vi "Process_Traces.vi"(8 "Process data parameters in":T1={"Stop loop"={"Settings changed?"=FALSE, "Stop?"=refnum}, "Button refs"={"Stop program"=refnum, "Save settings"=refnum, "DAQ mode"=refnum, "Reset settings"=refnum, "Apply settings"=refnum, "Reset MAS"=refnum, "Reset SLV"=refnum, "Local DBase?"=refnum, "Last value DBase"=FALSE, "Database"=refnum, "Calibration"=refnum, "Save settings 2"=refnum}, "Process messages"={"Process message mode"=enum."Error", "Slave data?"=FALSE, "Length get settings message"=0, "Delta time"=0.0, "Data_Filter"={"Filter_Data"=FALSE, "Use_Thresh"=FALSE, "Reduce data?"=FALSE}, "Time_difference_stack"=[], "Starting sec"=0, "Ending sec"=0, "Ending sec 2"=0, "MAS_Page_Thresh"=refnum, "SLV_Page_Thresh"=refnum, "Database"=refnum}, "Settings state"={"MAS locked?"=refnum, "SLV locked?"=refnum}, "Mode"={"Mode"=enum."Dialog", "Expert?"=FALSE, "Dialog?"=FALSE}, "Alignment parameters"=refnum, "Timer parameters"=refnum, "Files"={"Path config file"=path "", "Path def. ini file"=path "", "Path ini file 1"=path "", "Path ini file 2"=path "", "Path RBF file"=path ""}, "Time difference"=refnum, "Alignment"={"GEN_Page_Calibrate"=refnum, "MAS_Page_Gain"=refnum, "MAS_Page_Offset"=refnum, "SLV_Page_Gain"=refnum, "SLV_Page_Offset"=refnum, "MAS_Page_Common"=refnum, "SLV_Page_Common"=refnum}, "Page Statistics"=refnum}, 9 "Length":i32, 10 "Data in":u8[](array[numeric]), 11 "Master?":bool=TRUE) -> (1 "Cut off":i16[](array[numeric]), 2 "Data out":u8[](array[numeric]), 3 "Offset":i16[](array[numeric]))   [LabVIEW 2013]
uses:
  Controls/Stop_Loop.ctl
  Controls/Button_Refs.ctl
  Controls/Process_Message_Mode.ctl
  Controls/Process_Messages.ctl
  Controls/Settings_State.ctl
  Controls/Mode.ctl
  Controls/Files.ctl
  Controls/Process_Data_Parameters.ctl
  Controls/Page_Calibration.ctl
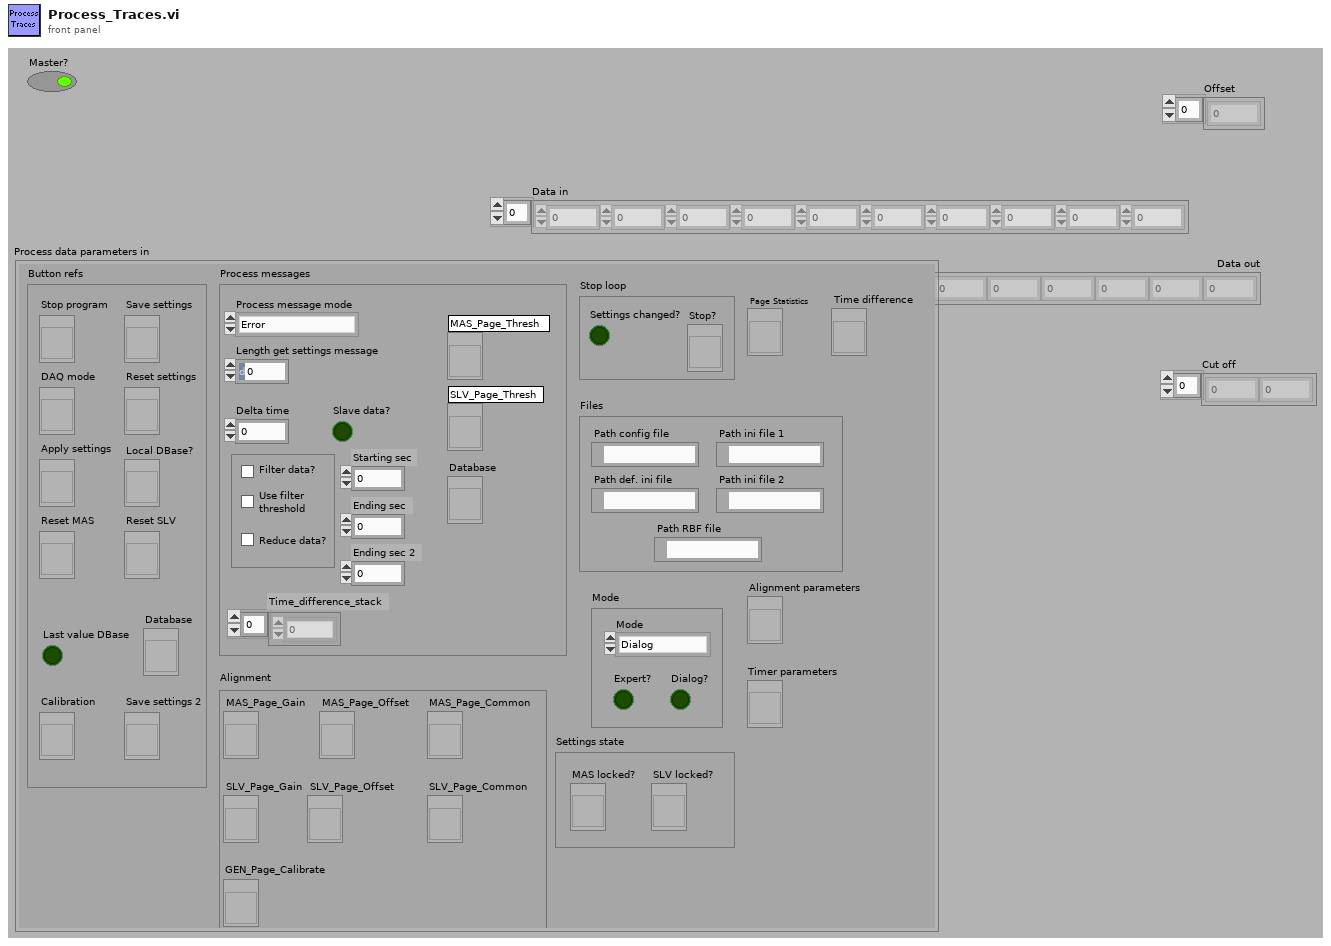
[diagram p1: front panel]
types:
  T1 = typedef "Process_Data_Parameters.ctl" = cluster{"Stop loop":T2, "Button refs":T3, "Process messages":T4, "Settings state":T6, "Mode":T7, "Alignment parameters":refnum<vi>, "Timer parameters":refnum<vi>, "Files":T8, "Time difference":refnum<vi>, "Alignment":T9, "Page Statistics":refnum<vi>}
  T2 = typedef "Stop_Loop.ctl" = cluster{"Settings changed?":bool, "Stop?":refnum<vi>}
  T3 = typedef "Button_Refs.ctl" = cluster{"Stop program":refnum<vi>, "Save settings":refnum<vi>, "DAQ mode":refnum<vi>, "Reset settings":refnum<vi>, "Apply settings":refnum<vi>, "Reset MAS":refnum<vi>, "Reset SLV":refnum<vi>, "Local DBase?":refnum<vi>, "Last value DBase":bool, "Database":refnum<vi>, "Calibration":refnum<vi>, "Save settings 2":refnum<vi>}
  T4 = typedef "Process_Messages.ctl" = cluster{"Process message mode":T5, "Slave data?":bool, "Length get settings message":i32, "Delta time":dbl, "Data_Filter":cluster{"Filter_Data":bool, "Use_Thresh":bool, "Reduce data?":bool}, "Time_difference_stack":u64[], "Starting sec":u64, "Ending sec":u64, "Ending sec 2":u64, "MAS_Page_Thresh":refnum<vi>, "SLV_Page_Thresh":refnum<vi>, "Database":refnum<vi>}
  T5 = typedef "Process_Message_Mode.ctl" = enum16{"Error", "Measurement data", "Comparator data", "One Second"}
  T6 = typedef "Settings_State.ctl" = cluster{"MAS locked?":refnum<vi>, "SLV locked?":refnum<vi>}
  T7 = typedef "Mode.ctl" = cluster{"Mode":enum8{"Stop", "Dialog", "Hisparc II", "Hisparc II DAQ", "Alignment"}, "Expert?":bool, "Dialog?":bool}
  T8 = typedef "Files.ctl" = cluster{"Path config file":path, "Path def. ini file":path, "Path ini file 1":path, "Path ini file 2":path, "Path RBF file":path}
  T9 = typedef "Page_Calibration.ctl" = cluster{"GEN_Page_Calibrate":refnum<vi>, "MAS_Page_Gain":refnum<vi>, "MAS_Page_Offset":refnum<vi>, "SLV_Page_Gain":refnum<vi>, "SLV_Page_Offset":refnum<vi>, "MAS_Page_Common":refnum<vi>, "SLV_Page_Common":refnum<vi>}
  T10 = cluster{"Filter_Data":bool, "Use_Thresh":bool, "Reduce data?":bool}
  T11 = cluster{"Ch1_Thres_Low":dbl, "Ch1_Thres_High":dbl, "Ch2_Thres_Low":dbl, "Ch2_Thres_High":dbl}
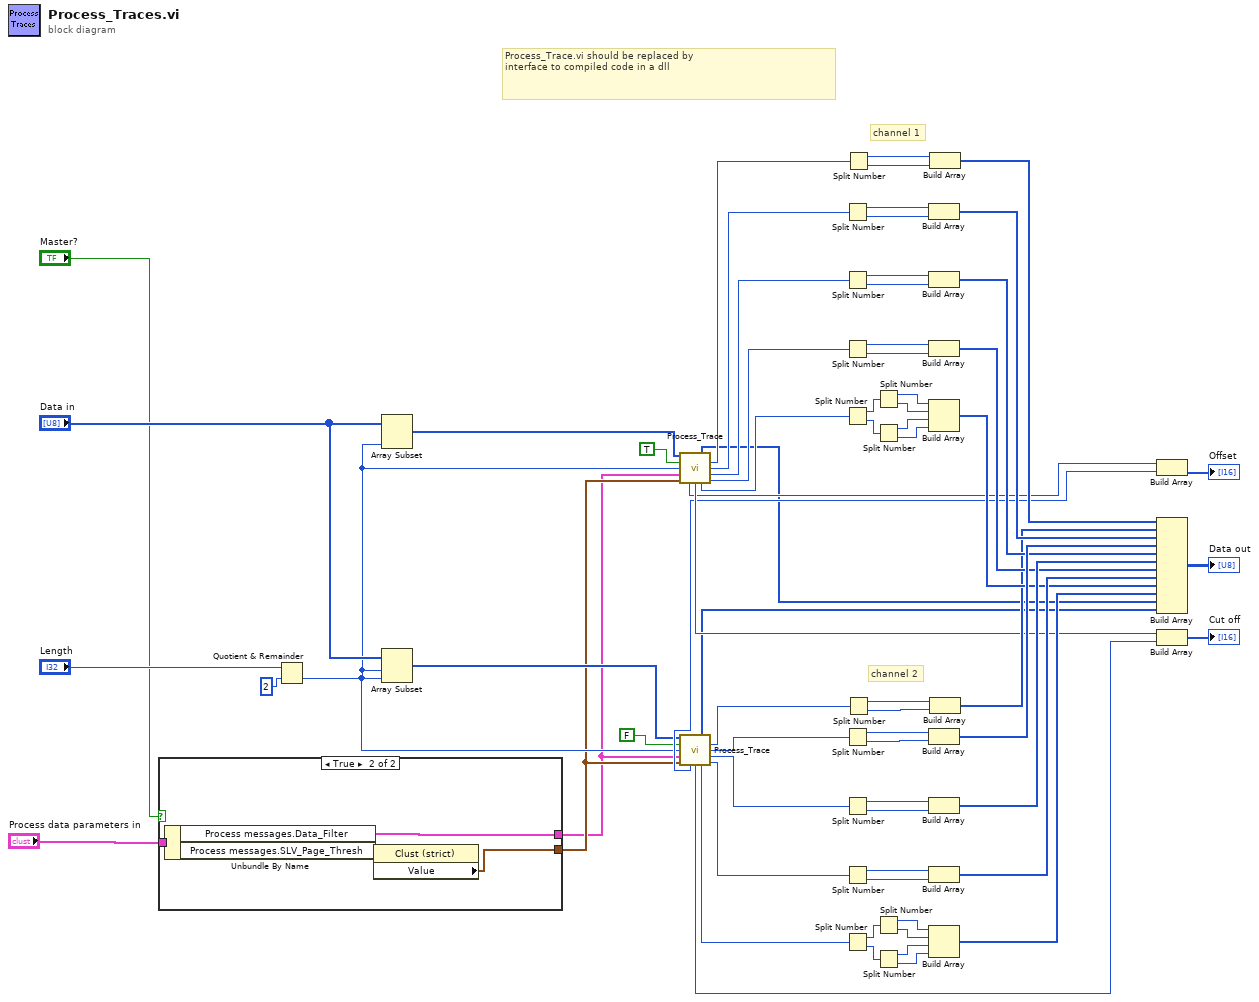
[diagram p0: block diagram]
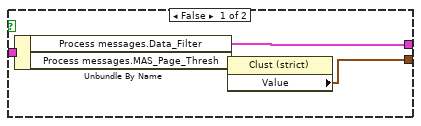
[diagram p2: hidden frame]
diagram:
  # "channel 1"
  # "channel 2"
  # "Process_Trace.vi should be replaced by\ninterface to compiled code in a dll"
  n1 = case shown="True" "Master?" {
    tunnel: "Process data parameters in" -> [w73 w77]
    tunnel: [w70 w74] -> w5
    tunnel: [w72 w76] -> w4
    frame False {
      n2 = Unbundle By Name(w73) -> ("Process messages.Data_Filter"=w72:T10, "Process messages.MAS_Page_Thresh"=w71:refnum<vi>)
      n3 = property class="Clust (strict)"(reference=w71) -> ("Value"=w70:T11)  [unwired: 1 in, 2 out]
    }
    frame True {
      n4 = Unbundle By Name(w77) -> ("Process messages.Data_Filter"=w76:T10, "Process messages.SLV_Page_Thresh"=w75:refnum<vi>)
      n5 = property class="Clust (strict)"(reference=w75) -> ("Value"=w74:T11)  [unwired: 1 in, 2 out]
    }
  }
  n6 = Quotient & Remainder(x="Length", y=2) -> (floor(x/y)=w8:i32)  [unwired: 1 out]
  n7 = Array Subset(array="Data in", length=w8) -> (w10:u8[])  [unwired: 1 in]
  n8 = Array Subset(array="Data in", index=w8, length=w8) -> (w9:u8[])
  n9 = call "Process_Trace.vi"("Data in"=w10, "Channel 1?"=TRUE, "Length"=w8, "Data_Filter"=w4, "M-Thresholds"=w5) -> ("Data out (8 bits)"=w1:u8[], "Standard deviation"=w24:i16, "Baseline"=w22:i16, "Number of peaks"=w20:i16, "Offset"=w12:i16, "Cut off"=w14:i16, "Integral"=w16:i32, "Pulse height"=w18:i16)  [unwired: 1 in, 2 out]
  n10 = call "Process_Trace.vi"("Data in"=w9, "Channel 1?"=FALSE, "Length"=w8, "Data_Filter"=w4, "M-Thresholds"=w5) -> ("Data out (8 bits)"=w2:u8[], "Standard deviation"=w23:i16, "Baseline"=w21:i16, "Number of peaks"=w19:i16, "Offset"=w11:i16, "Cut off"=w13:i16, "Integral"=w15:i32, "Pulse height"=w17:i16)  [unwired: 1 in, 2 out]
  n11 = Split Number(x=w22) -> (hi(x)=w40:u8, lo(x)=w39:u8)
  n12 = Split Number(x=w20) -> (hi(x)=w38:u8, lo(x)=w37:u8)
  n13 = Split Number(x=w18) -> (hi(x)=w36:u8, lo(x)=w35:u8)
  n14 = Split Number(x=w16) -> (hi(x)=w60:u16, lo(x)=w59:u16)
  n15 = Split Number(x=w21) -> (hi(x)=w46:u8, lo(x)=w45:u8)
  n16 = Split Number(x=w19) -> (hi(x)=w44:u8, lo(x)=w43:u8)
  n17 = Split Number(x=w17) -> (hi(x)=w42:u8, lo(x)=w41:u8)
  n18 = Split Number(x=w15) -> (hi(x)=w66:u16, lo(x)=w65:u16)
  n19 = Split Number(x=w24) -> (hi(x)=w32:u8, lo(x)=w31:u8)
  n20 = Split Number(x=w23) -> (hi(x)=w30:u8, lo(x)=w29:u8)
  n21 = Split Number(x=w60) -> (hi(x)=w58:u8, lo(x)=w57:u8)
  n22 = Split Number(x=w59) -> (hi(x)=w56:u8, lo(x)=w55:u8)
  n23 = Split Number(x=w66) -> (hi(x)=w64:u8, lo(x)=w63:u8)
  n24 = Split Number(x=w65) -> (hi(x)=w62:u8, lo(x)=w61:u8)
  n25 = Build Array(w40, w39) -> (w51:u8[])
  n26 = Build Array(w38, w37) -> (w49:u8[])
  n27 = Build Array(w36, w35) -> (w47:u8[])
  n28 = Build Array(w58, w57, w56, w55) -> (w48:u8[])
  n29 = Build Array(w46, w45) -> (w53:u8[])
  n30 = Build Array(w44, w43) -> (w54:u8[])
  n31 = Build Array(w42, w41) -> (w50:u8[])
  n32 = Build Array(w64, w63, w62, w61) -> (w52:u8[])
  n33 = Build Array(w32, w31) -> (w28:u8[])
  n34 = Build Array(w30, w29) -> (w27:u8[])
  n35 = Build Array(w12, w11) -> (→"Offset":i16[])
  n36 = Build Array(w28, w27, w51, w53, w49, w54, w47, w50, w48, w52, w1, w2) -> (→"Data out":u8[][])
  n37 = Build Array(w14, w13) -> (→"Cut off":i16[])
